vi "Write Firmware.vi"(0 "Device":T5, 2 "Handle":u32, 5 "Firmware data":u8[](array[numeric]), 11 "error in (no error)":errorcluster) -> (4 "Result":u32, 6 "nSTATUS":bool, 10 "CONF_DONE":bool, 15 "error out":errorcluster)   [LabVIEW 2010]
uses:
  Controls/SpiDevice.ctl
panel:
  in  "Data Control":T1
  in  "Init Condition":T2 {"Chip Select Pin" items=["ADBUS3 Chip Select", "ADBUS4 GPIOL1", "ADBUS5 GPIOL2", "ADBUS6 GPIOL3", "ADBUS7 GPIOL4"]}
  in  "High Output Pins":T3
  in  "Wait Data Write":T4
  out "nCONFIG":bool
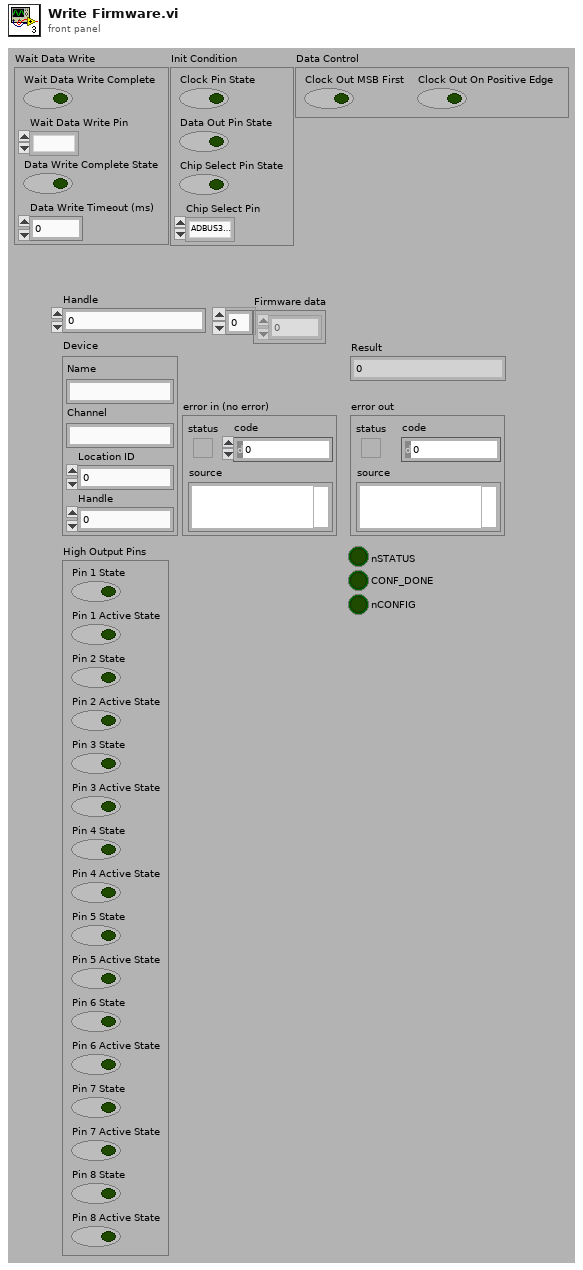
[diagram p1: front panel]
types:
  T1 = cluster{"Clock Out MSB First":bool, "Clock Out On Positive Edge":bool}
  T2 = cluster{"Clock Pin State":bool, "Data Out Pin State":bool, "Chip Select Pin State":bool, "Chip Select Pin":u16}
  T3 = cluster{"Pin 1 State":bool, "Pin 1 Active State":bool, "Pin 2 State":bool, "Pin 2 Active State":bool, "Pin 3 State":bool, "Pin 3 Active State":bool, "Pin 4 State":bool, "Pin 4 Active State":bool, "Pin 5 State":bool, "Pin 5 Active State":bool, "Pin 6 State":bool, "Pin 6 Active State":bool, "Pin 7 State":bool, "Pin 7 Active State":bool, "Pin 8 State":bool, "Pin 8 Active State":bool}
  T4 = cluster{"Wait Data Write Complete":bool, "Wait Data Write Pin":u16, "Data Write Complete State":bool, "Data Write Timeout (ms)":u32}
  T5 = typedef "SpiDevice.ctl" = cluster{"Name":string, "Channel":string, "Location ID":u32, "Handle":u32}
  T6 = cluster{"[0]":bool, "[1]":bool, "[2]":bool, "[3]":bool, "[4]":bool, "[5]":bool, "[6]":bool, "[7]":bool, "[8]":bool}
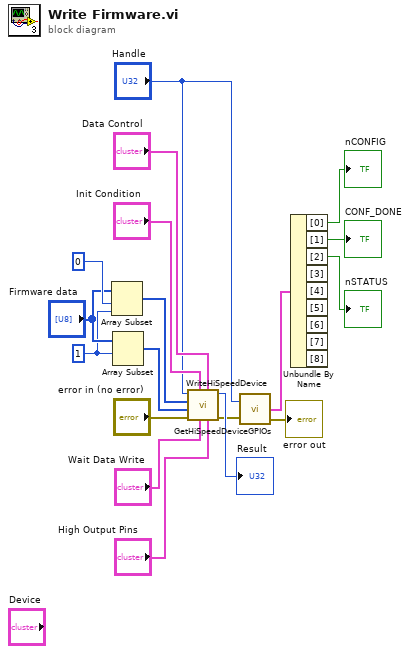
[diagram p0: block diagram]
diagram:
  w3 = 1 ("length")
  n1 = Array Subset(array="Firmware data", index=0, length=w3) -> (w5:u8[])
  n2 = Array Subset(array="Firmware data", index=w3) -> (w2:u8[])  [unwired: 1 in]
  n3 = call "WriteHiSpeedDevice.vi"("High Output Pins"="High Output Pins", "Data Control"="Data Control", "Wait Data Write"="Wait Data Write", "Init Condition"="Init Condition", "error in (no error)"="error in (no error)", "Data Buffer"=w2, "Control Buffer"=w5, "Handle"="Handle") -> ("error out"=w11:errorcluster, "Result"=→"Result":u32)  [unwired: 2 in]
  n4 = call "GetHiSpeedDeviceGPIOs.vi"("Handle"="Handle", "error in (no error)"=w11) -> ("High IO Values"=w9:T6, "error out"=→"error out":errorcluster)  [unwired: 1 out]
  n5 = Unbundle By Name(w9) -> ("[0]"=→"nCONFIG":bool, "[1]"=→"CONF_DONE":bool, "[2]"=→"nSTATUS":bool)  [unwired: 6 out]
